vi "MoveVel.vi"(0 "OBJ":dbl[](array[numeric]), 11 "error in (no error)":errorcluster) -> (15 "error out":errorcluster)   [LabVIEW 2019]
panel:
  in  "stop":bool
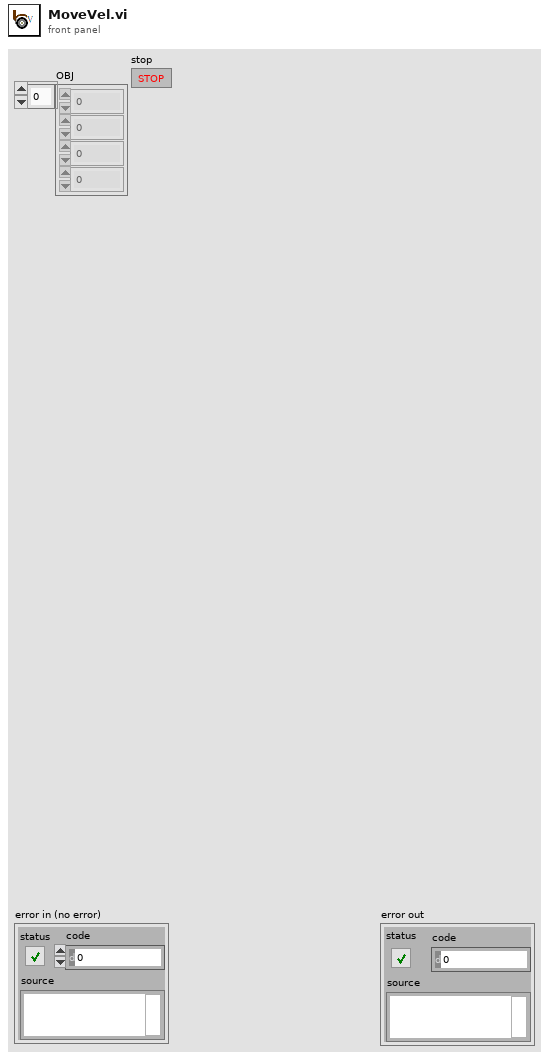
[diagram p1: front panel]
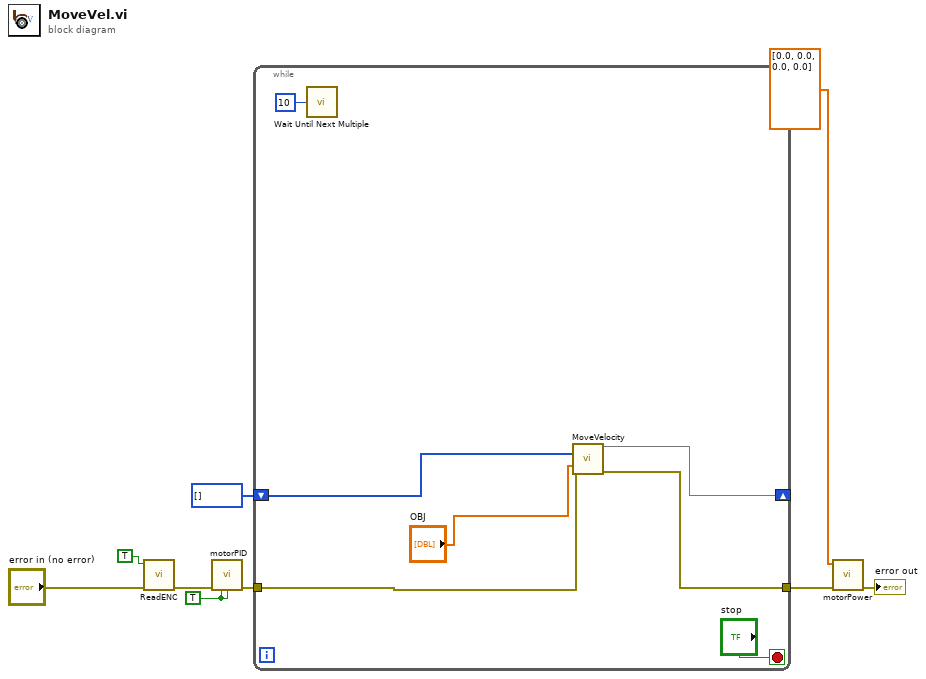
[diagram p0: block diagram]
diagram:
  w2 = TRUE ("EncRst")
  n1 = call "ReadENC.vi"("error in (no error)"="error in (no error)", "Reset"=TRUE) -> ("error out"=w3:errorcluster)  [unwired: 8 in, 1 out]
  n2 = call "motorPID.vi"("error in (no error)"=w3, "reinitialize? (F)"=w2, "EncRst"=w2) -> ("error out"=w8:errorcluster)  [unwired: 9 in, 3 out]
  n3 = while {
    tunnel: w8 -> [w15]
    tunnel: [w14] -> w7
    shift-right: [w12] -> _
    shift-left: i32[] [] ("ENC") -> [w11]
    stop <- "stop" stop-if-true
    n4 = call "Wait Until Next Multiple"("Count(mSec)"=u32 10) -> ()  [unwired: 1 out]
    n5 = call "MoveVelocity.vi"(5:w11, "OBJ"="OBJ", "error in (no error)"=w15) -> (4:w12, "error out"=w14:errorcluster)  [unwired: 8 in, 3 out]
  }
  n6 = call "motorPower.vi"("error in (no error)"=w7, "DC_Pwr"=dbl[] [0.0, 0.0, 0.0, 0.0]) -> ("error out"=→"error out":errorcluster)  [unwired: 9 in]
